vi "VI Main 1.0.vi"() -> ()   [LabVIEW 2014]
uses:
  <vilib>/Analysis/NI_AALPro.lvlib
panel:
  in  "Reset":bool
  in  "Start":bool
  in  "stop":bool
  out "intercept":dbl format="%_4g"
  out "Waveform Chart":dbl(graph)=1498.7145698358406
  out "Res. (ohm)":dbl=1498.7145698358406 format="%#.5g"
  out "XY Graph":cluster{dbl[], "Best Linear Fit":dbl[]}[](graph)
  in  "sense range":i32(slide)
  in  "stop (V)":dbl=5.0 format="%.4f"
  in  "source compliance (A)":dbl=0.01 format="%.4f"
  in  "direction":i32(slide)
  in  "spacing":i32(slide)
  in  "ranging":i32(slide)
  in  "start (V)":dbl step=1.0 format="%.2p"
  in  "number of points":i32=20 min=1 max=2500 step=1
  in  "speed":i32(slide)=2
  in  "source protection (V)":dbl=2.0 format="%.4f"
  out "status":i32 format="%.0x"
  in  "resource name 2":string="GPIB4::24::INSTR"
  in  "resource name":string="ASRL4::INSTR"
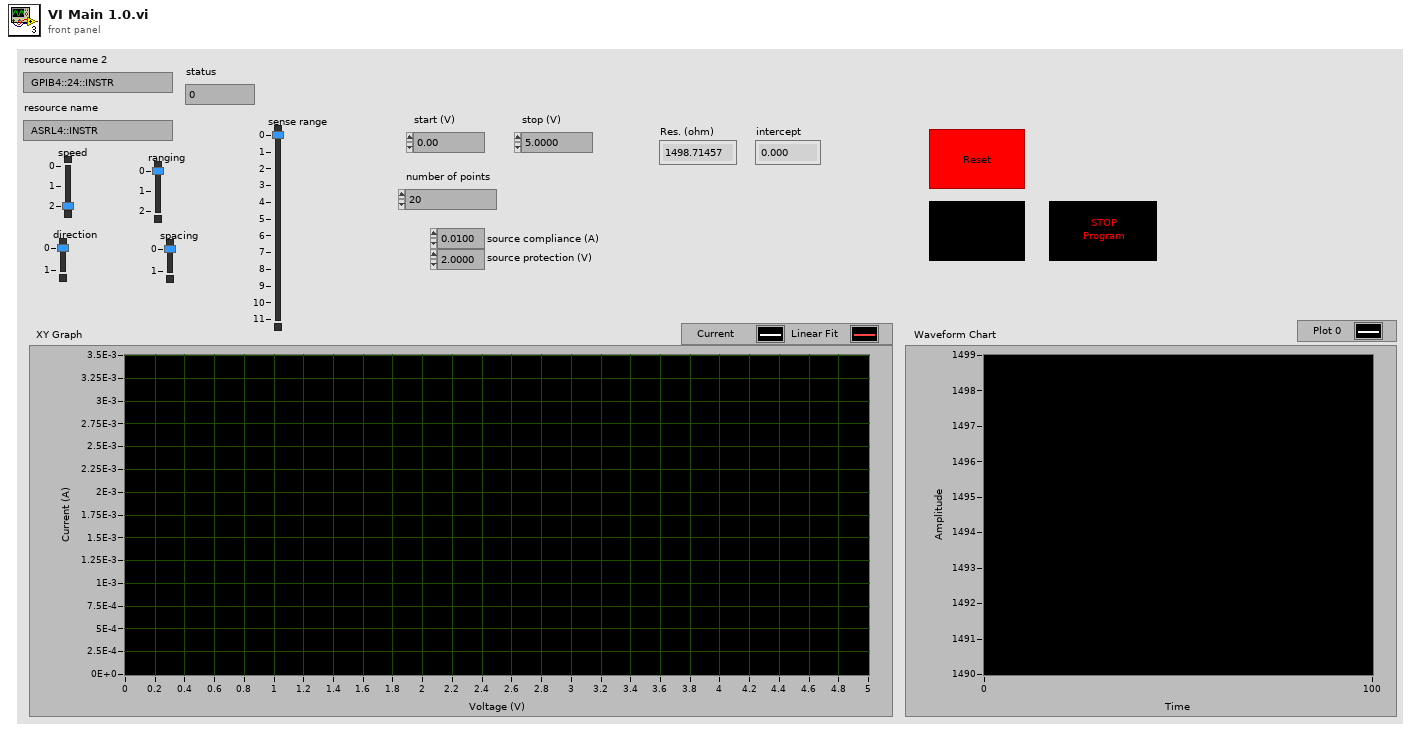
[diagram p1: front panel]
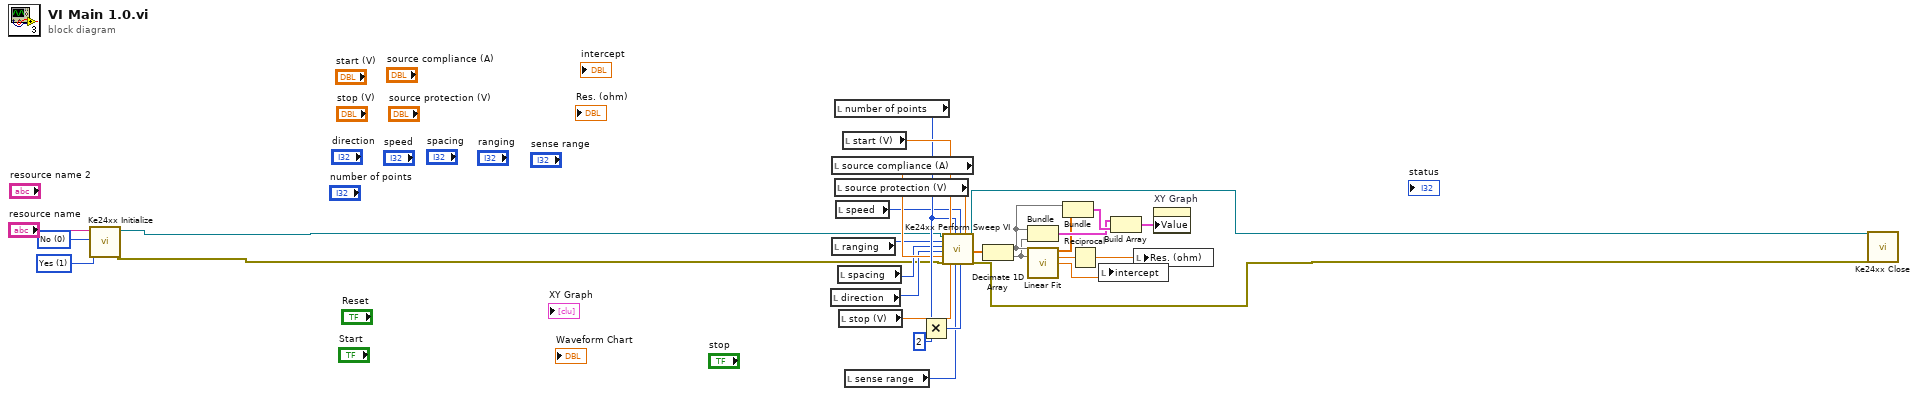
[diagram p0: block diagram]
diagram:
  w28 = u16 1 items=["Yes"=1, "No"=0] ("id query")
  w29 = u16 0 items=["Yes"=1, "No"=0] ("reset device")
  n1 = call <instrlib>:"Ke24xx Initialize.vi"("reset device"=w29, "id query"=w28, "resource name"="resource name") -> ("error out"=w1:errorcluster, "instrument handle out"=w2:refnum<visa-resource-name>)  [unwired: 6 in, 1 out]
  n2 = local read "direction"() -> (w3:i32)
  n3 = local read "source compliance (A)"() -> (w8:dbl)
  n4 = local read "ranging"() -> (w5:i32)
  n5 = local read "number of points"() -> (w11:i32)
  n6 = local read "source protection (V)"() -> (w7:dbl)
  n7 = local read "speed"() -> (w6:i32)
  n8 = local read "spacing"() -> (w4:i32)
  n9 = local read "stop (V)"() -> (w13:dbl)
  n10 = local read "start (V)"() -> (w14:dbl)
  n11 = local read "sense range"() -> (w9:i32)
  n12 = Multiply(x=w11, y=2) -> (x*y=w10:i32)
  n13 = call <instrlib>:"Ke24xx Perform Sweep VI.vi"("instrument handle"=w2, "ranging"=w5, "spacing"=w4, "direction"=w3, "source compliance"=w8, "error in (no error)"=w1, "start"=w14, "stop"=w13, "number of points"=w11, "sense range"=w9, "speed"=w6, "size of reading"=w10, "source protection"=w7) -> ("instrument handle out"=w26:refnum<visa-resource-name>, "out"=w18:dbl[], "error out"=w25:errorcluster)  [unwired: 3 in, 1 out]
  n14 = Decimate 1D Array(w18) -> (w22:dbl[], w19:dbl[])
  n15 = Bundle(w22, w19) -> (w23:cluster{dbl[], dbl[]})  [unwired: 1 in]
  n16 = call <vilib>:"Linear Fit.vi"("Y"=w19, "X"=w22) -> ("Best Linear Fit"=w21:dbl[], "slope"=w20:dbl, "intercept"=w17:dbl)  [unwired: 9 in, 2 out]
  n17 = Bundle(w22, "Best Linear Fit"=w21) -> (w24:cluster{dbl[], "Best Linear Fit":dbl[]})  [unwired: 1 in]
  n18 = Reciprocal(x=w20) -> (1/x=w16:dbl)
  n19 = local write "intercept"(w17) -> ()
  n20 = Build Array(w23, w24) -> (w15:cluster{dbl[], "Best Linear Fit":dbl[]}[])
  n21 = local write "Res. (ohm)"(w16) -> ()
  n22 = property on="XY Graph" class="XYGraph (strict)"("Value"=w15) -> ()  [unwired: 2 in, 2 out]
  n23 = call <instrlib>:"Ke24xx Close.vi"("error in (no error)"=w25, "instrument handle"=w26) -> ()  [unwired: 8 in, 2 out]
